vi "Main.vi"() -> ()   [LabVIEW 2017]
doc: "The myRIO Project template acquires acceleration data from the onboard accelerometer and displays the changes of acceleration values in a waveform chart."
panel:
  in  "Stop Button":bool
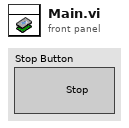
[diagram p1: front panel]
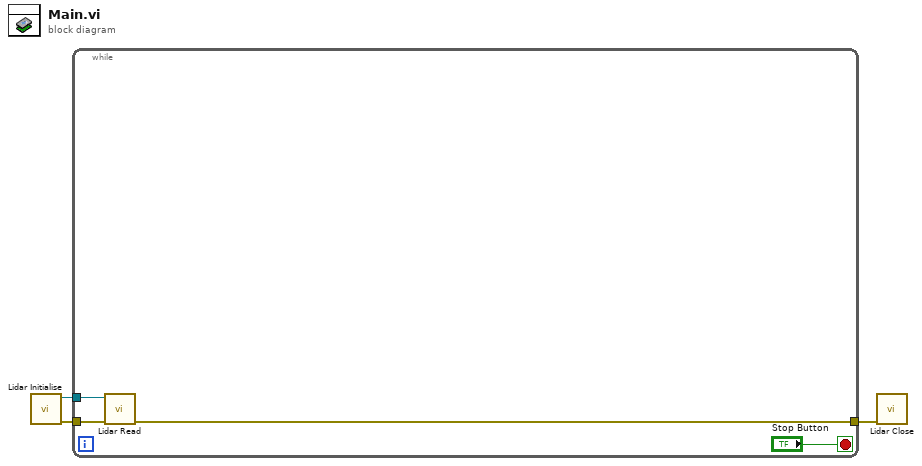
[diagram p0: block diagram]
diagram:
  n1 = call "Lidar Initialise.vi"() -> ("error out"=w1:errorcluster, "VISA resource name out"=w2:refnum<visa-resource-name>)  [unwired: 10 in]
  n2 = while {
    tunnel: [w7] -> w3
    tunnel: w2 -> [w6]
    tunnel: w1 -> [w5]
    stop <- "Stop Button" stop-if-true
    n3 = call "Lidar Read.vi"("error in (no error)"=w5, "VISA resource name"=w6) -> ("error out"=w7:errorcluster)  [unwired: 4 in, 4 out]
  }
  n4 = call "Lidar Close.vi"("error in (no error)"=w3) -> ()  [unwired: 10 in, 1 out]
